vi "lasersSetFrequencies_IV.vi"(0 "VISA Refnum in":refnum<visa-resource-name>, 5 "f-res (Hz)":dbl, 11 "error in (no error)":errorcluster) -> (4 "405 f (Hz)":i32, 6 "532 f (Hz)":i32, 8 "662 f (Hz)":i32, 10 "785 f (Hz)":i32, 15 "error out":errorcluster)   [LabVIEW 2011]
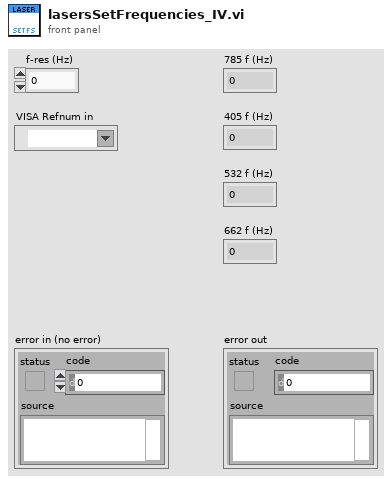
[diagram p1: front panel]
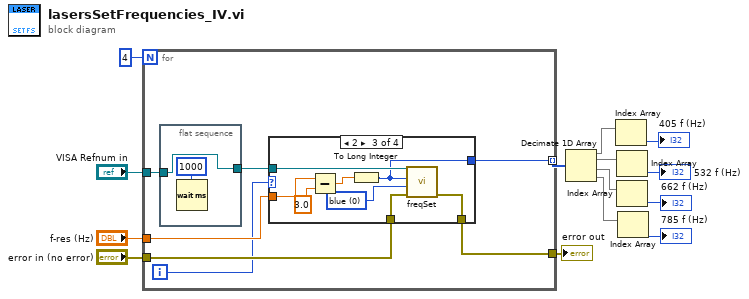
[diagram p0: block diagram]
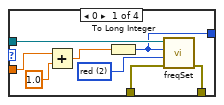
[diagram p2: hidden frame]
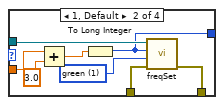
[diagram p3: hidden frame]
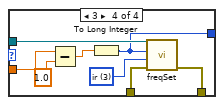
[diagram p4: hidden frame]
diagram:
  n1 = for {
    N: 4 ("Number of Lasers") -> [_]
    tunnel: [w21] -> w5
    tunnel: "error in (no error)" -> [w20]
    tunnel: "VISA Refnum in" -> [w17]
    tunnel: "f-res (Hz)" -> [w19]
    tunnel: [w15] -> w6 mode=indexing
    i -> [w18]
    n2 = flat-sequence {
      tunnel: w17 -> [w22]
      tunnel: [w22] -> w16
      frame #0 {
        n3 = Wait (ms)(milliseconds to wait=u32 1000) -> ()  [unwired: 1 out]
      }
    }
    n4 = case shown="2" w18 {
      tunnel: [w31 w39 w47 w55] -> w21
      tunnel: w20 -> [w29 w36 w44 w53]
      tunnel: w16 -> [w28 w35 w43 w52]
      tunnel: w19 -> [w24 w33 w41 w50]
      tunnel: [w27 w32 w40 w49] -> w15
      frame 0 {
        w30 = u16 2 items=["blue", "green", "red"] ("laser")
        n5 = Add(x=w24, y=1.0) -> (x+y=w26:dbl)
        n6 = To Long Integer(number=w26) -> (32bit integer=w27:i32)
        n7 = call "freqSet.vi"("error in (no error)"=w29, "laser"=w30, "Freq, Hz (1370)"=w27, "Teensy Port"=w28) -> ("error out"=w31:errorcluster)  [unwired: 6 in, 1 out]
      }
      frame 1, Default {
        w38 = u16 1 items=["blue", "green", "red"] ("laser")
        n8 = Add(x=w33, y=3.0) -> (x+y=w34:dbl)
        n9 = To Long Integer(number=w34) -> (32bit integer=w32:i32)
        n10 = call "freqSet.vi"("error in (no error)"=w36, "laser"=w38, "Freq, Hz (1370)"=w32, "Teensy Port"=w35) -> ("error out"=w39:errorcluster)  [unwired: 6 in, 1 out]
      }
      frame 2 {
        w46 = u16 0 items=["blue", "green", "red"] ("laser")
        n11 = Subtract(x=w41, y=3.0) -> (x-y=w42:dbl)
        n12 = To Long Integer(number=w42) -> (32bit integer=w40:i32)
        n13 = call "freqSet.vi"("error in (no error)"=w44, "laser"=w46, "Freq, Hz (1370)"=w40, "Teensy Port"=w43) -> ("error out"=w47:errorcluster)  [unwired: 6 in, 1 out]
      }
      frame 3 {
        w48 = u16 3 items=["blue", "green", "red", "ir"] ("laser")
        n14 = Subtract(x=w50, y=1.0) -> (x-y=w51:dbl)
        n15 = To Long Integer(number=w51) -> (32bit integer=w49:i32)
        n16 = call "freqSet.vi"("error in (no error)"=w53, "laser"=w48, "Freq, Hz (1370)"=w49, "Teensy Port"=w52) -> ("error out"=w55:errorcluster)  [unwired: 6 in, 1 out]
      }
    }
  }
  "error out" <- w5
  n17 = Decimate 1D Array(w6) -> (w7:i32[], w9:i32[], w10:i32[], w13:i32[])
  n18 = Index Array(array=w7) -> (element=→"405 f (Hz)":i32)  [unwired: 1 in]
  n19 = Index Array(array=w9) -> (element=→"532 f (Hz)":i32)  [unwired: 1 in]
  n20 = Index Array(array=w10) -> (element=→"662 f (Hz)":i32)  [unwired: 1 in]
  n21 = Index Array(array=w13) -> (element=→"785 f (Hz)":i32)  [unwired: 1 in]
